vi "Drop Message Core.vi"(11 "Ping Msg in":refnum<class "Ping Msg.lvclass">) -> ()   [LabVIEW 2020, in "Actor Framework.lvlib" / "Ping Msg.lvclass"]
doc: "(<B>Filename</B>: Actor Framework.lvlib:Message.lvclass:Drop Message Core.vi)\n\nDefines what a message does if it is in the message queue when the queue is released. At this point, the actor has shut down, so it will never process the message.\n\nBy default, this method does nothing. A child class may override it to define behavior. National Instruments provides the Reply Msg class to override this method. This class releases its internal queue, which causes any caller of the Send Message and Wait For Response method to stop waiting and return an error."
uses:
  Ping Msg.lvclass
  Ping Msg.lvclass/Ping Msg.ctl
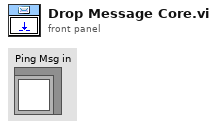
[diagram p1: front panel]
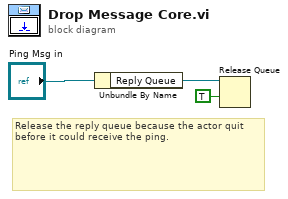
[diagram p0: block diagram]
diagram:
  # "Release the reply queue because the actor quit before it could receive the ping."
  n1 = Unbundle By Name("Ping Msg in") -> ("Reply Queue"=w1:refnum<queue>)
  n2 = Release Queue(queue=w1, force destroy? (F)=TRUE) -> ()  [unwired: 1 in, 3 out]
